vi "Image Acquisition.vi"(7 "Save File Path":path, 8 "Error In":errorcluster, 9 "Image Index In":dbl, 10 "Record Button":bool) -> (0 "Error Out":errorcluster, 1 "Image Index Out":dbl, 2 "Right Image":T2(plugin-control), 3 "Left Image":T2(plugin-control), 4 "Gauge":cluster{dbl, dbl}(knob) scale=0.0..50.0, 5 "Time Stamp":timestamp)   [LabVIEW 2012]
panel:
  out "Image Type":T1 items=["Grayscale (U8)", "Grayscale (I16)", "Grayscale (SGL)", "Complex (CSG)", "RGB (U32)", "HSL (U32)", "RGB (U64)", "Grayscale (U16)"]
  out "Y Resolution":i32
  out "X Resolution":i32
  out "RGB":u32[][](graph)
  out "HSV":u32[][](graph)
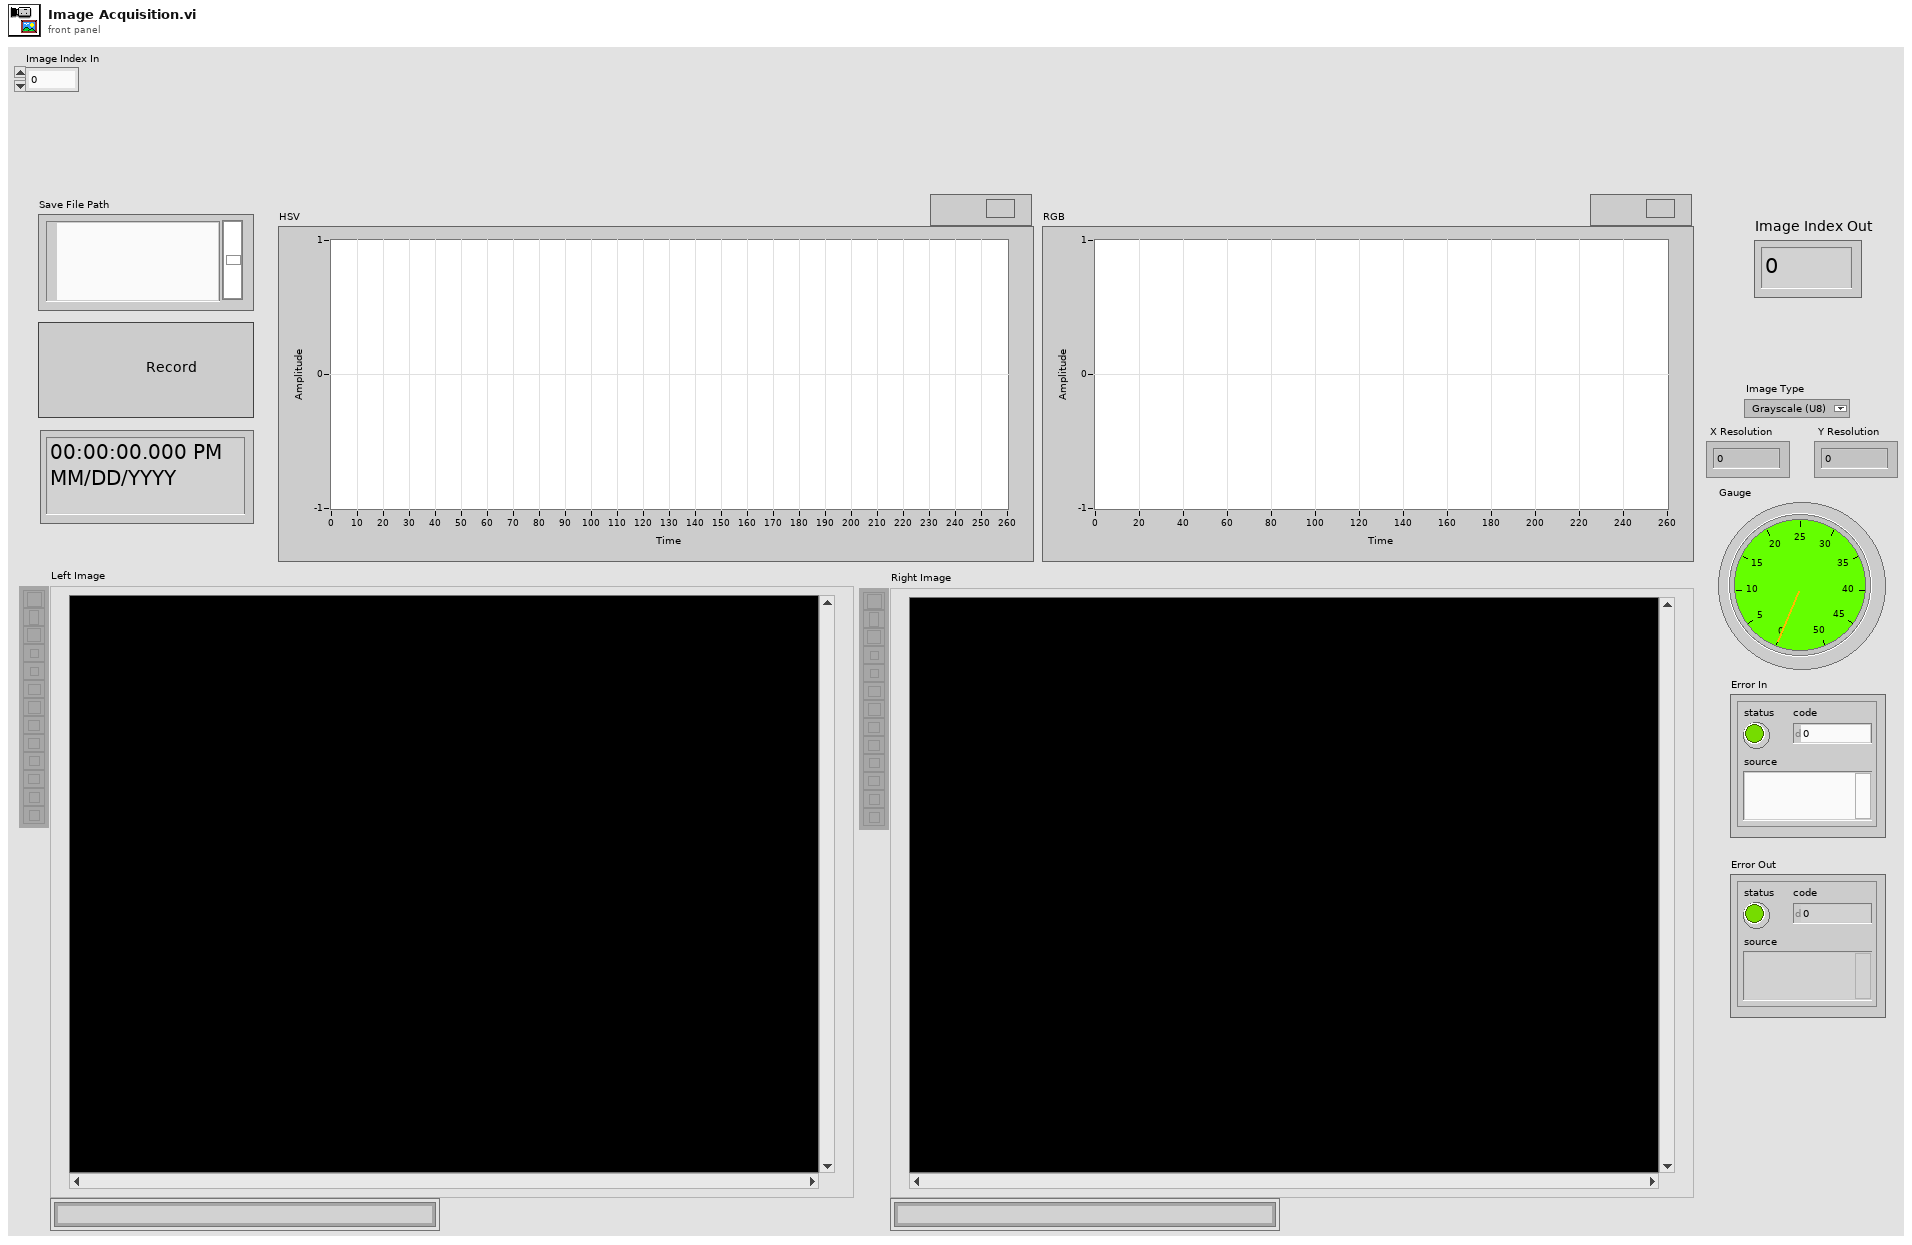
[diagram p1: front panel]
types:
  T1 = typedef "Image Type" = u32
  T2 = typedef "IMAQ Image.ctl" = refnum<image>
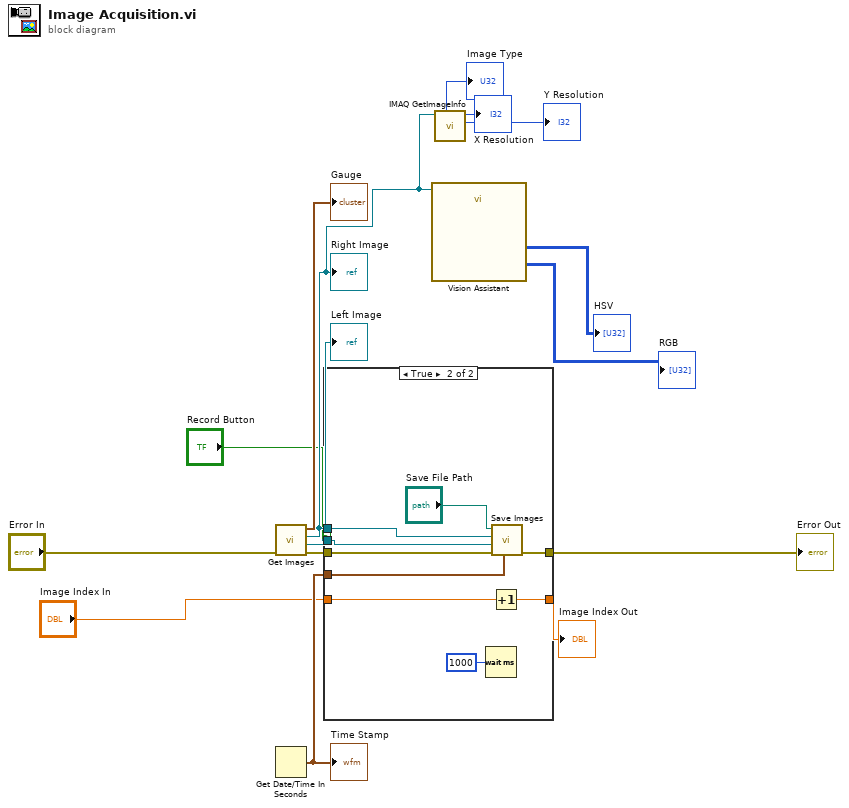
[diagram p0: block diagram]
diagram:
  n1 = call "Get Images.vi"("error in"="Error In") -> ("error out"=w12:errorcluster, "Left Image out"=w10:T2, "Right Image out"=w7:T2, "Gauge"=→"Gauge":cluster{dbl, dbl})  [unwired: 7 in]
  "Left Image" <- w10
  "Right Image" <- w7
  n2 = Get Date/Time In Seconds() -> (seconds since 1Jan1904=w14:timestamp)
  "Time Stamp" <- w14
  n3 = case shown="True" "Record Button" {
    tunnel: w14 -> [_ w26]
    tunnel: [w17 w25] -> w13
    tunnel: w12 -> [w16 w24]
    tunnel: w10 -> [_ w23]
    tunnel: w7 -> [_ w22]
    tunnel: "Image Index In" -> [w17 w21]
    tunnel: [w16 w18] -> w1
    frame False {
    }
    frame True {
      n4 = Wait (ms)(milliseconds to wait=u32 1000) -> ()  [unwired: 1 out]
      n5 = Increment(x=w21) -> (x+1=w25:dbl)
      n6 = call "Save Images.vi"("Time Stamp"=w26, "error in (no error)"=w24, "Left Image"=w23, "Right Image"=w22, "Save File Path"="Save File Path") -> ("error out"=w18:errorcluster)  [unwired: 6 in]
    }
  }
  "Error Out" <- w1
  "Image Index Out" <- w13
  n7 = call "Vision Assistant"("Image In"=w7) -> ("Histogram (Histogram 1)"=→"HSV":u32[][], "Histogram (Histogram 2)"=→"RGB":u32[][])  [unwired: 23 in, 2 out]
  n8 = call "IMAQ GetImageInfo"("Image"=w7) -> ("Y Resolution"=→"Y Resolution":i32, "X Resolution"=→"X Resolution":i32, "Image Type"=→"Image Type":T1)  [unwired: 3 in, 5 out]
